vi "check limits.vi"(8 "error in (no error)":errorcluster, 11 "Motor in":refnum<class "Motor.lvclass">) -> (0 "error out":errorcluster, 1 "Negetive_L":bool, 2 "Positive_L":bool, 3 "Motor out":refnum<class "Motor.lvclass">)   [LabVIEW 2019, in "Motor.lvclass"]
uses:
  Motor.lvclass
  Motor.lvclass/Motor.ctl
  Motor Serial class/Serial.lvclass
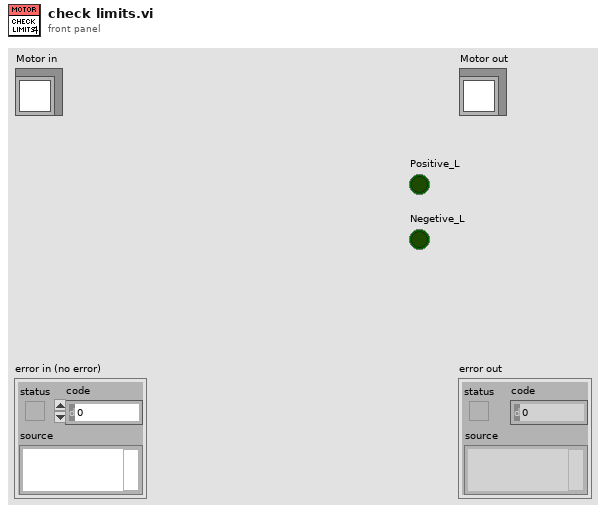
[diagram p1: front panel]
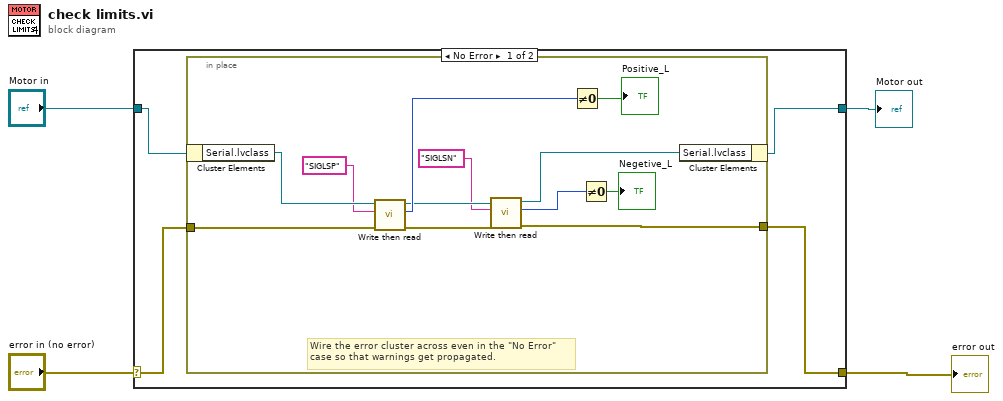
[diagram p0: block diagram]
diagram:
  n1 = case shown="No Error" "error in (no error)" {
    selector: "error in (no error)" -> [w5 w22]
    tunnel: [w6 w22] -> w3
    tunnel: [w7 w21] -> w1
    tunnel: "Motor in" -> [w8 w21]
    frame No Error {
      n2 = in-place {
        in-place-border: [w13] -> w6
        in-place-border: w5 -> [w11]
        # "Wire the error cluster across even in the \"No Error\"\ncase so that warnings get propagated."
        n3 = in-place-cluster #1(w8) -> ("Serial.lvclass"=w12:refnum<class "Serial.lvclass">)
        n4 = call "Write then read.vi"("error in (no error)"=w11, "TX Data"="SIGLSP" ("string"), "Motor_Serial in"=w12) -> ("error out"=w17:errorcluster, "RX Data"=w18:i32, "Motor_Serial out"=w16:refnum<class "Serial.lvclass">)  [unwired: 5 in]
        n5 = call "Write then read.vi"("error in (no error)"=w17, "TX Data"="SIGLSN" ("string"), "Motor_Serial in"=w16) -> ("error out"=w13:errorcluster, "RX Data"=w15:i32, "Motor_Serial out"=w14:refnum<class "Serial.lvclass">)  [unwired: 5 in]
        n6 = Not Equal To 0?(x=w18) -> (x != 0?=→"Positive_L":bool)
        n7 = Not Equal To 0?(x=w15) -> (x != 0?=→"Negetive_L":bool)
        n8 = in-place-cluster #1("Serial.lvclass"=w14) -> (w7:refnum<class "Motor.lvclass">)
      }
    }
    frame Error {
    }
  }
  "error out" <- w3
  "Motor out" <- w1
